vi "9217_Config to Channels.vi"(8 "error in (no error)":errorcluster, 11 "_9217 Config Data":T2={"Conversion Time"=0, "Degree Range"=[], "RTD_Type"=[1], "RTD_A"=[], "RTD_B"=[], "RTD_C"=[], "RTD_Ro"=[]} {"Conversion Time" items=["200 ms", "2.5 ms"]; "Degree Range" items=["Raw Ohms", "Degrees Kelvin", "Degrees Celsius", "Degrees Fahrenheit", "Degrees Rankine"]; "RTD_Type" items=["TCR3851"=1, "TCR3750"=2, "TCR3916"=3, "TCR3920"=4, "TCR3911"=5, "TCR3928"=6, "Custom"=0]}) -> (0 "error out":errorcluster, 2 "Conversion Time":u16(ring) items=["200 ms", "2.5 ms"], 3 "Channels":T1(array[cluster]))   [LabVIEW 2011, in "Modules.lvlib" / "9217.lvclass"]
uses:
  9217.lvclass
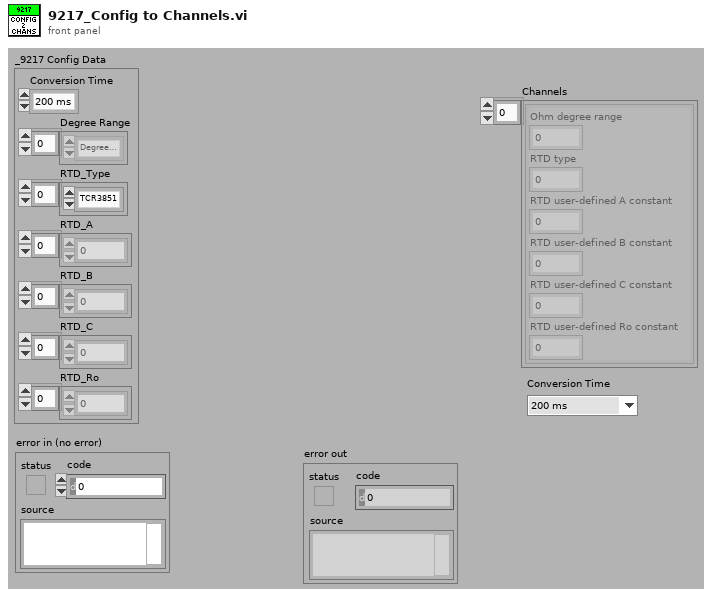
[diagram p1: front panel]
types:
  T1 = cluster{"Ohm degree range":u32, "RTD type":u32, "RTD user-defined A constant":dbl, "RTD user-defined B constant":dbl, "RTD user-defined C constant":dbl, "RTD user-defined Ro constant":dbl}[]
  T2 = cluster{"Conversion Time":u16, "Degree Range":u8[], "RTD_Type":u8[], "RTD_A":dbl[], "RTD_B":dbl[], "RTD_C":dbl[], "RTD_Ro":dbl[]}
  T3 = cluster{"Ohm degree range":u32, "RTD type":u32, "RTD user-defined A constant":dbl, "RTD user-defined B constant":dbl, "RTD user-defined C constant":dbl, "RTD user-defined Ro constant":dbl}
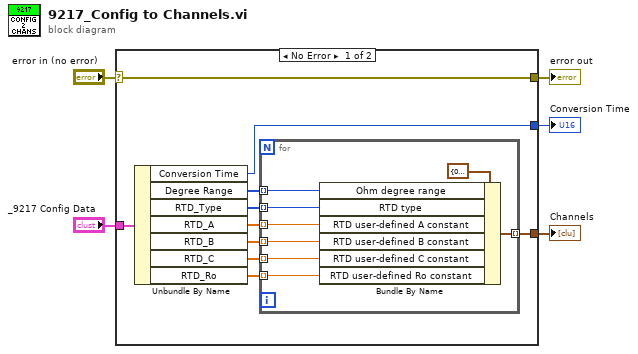
[diagram p0: block diagram]
diagram:
  n1 = case shown="No Error" "error in (no error)" {
    selector: "error in (no error)" -> [w15 w24]
    tunnel: [w15 w24] -> w4
    tunnel: "_9217 Config Data" -> [w14 _]
    tunnel: [w12 _] -> w2
    tunnel: [w6 _] -> w1
    frame No Error {
      n2 = Unbundle By Name(w14) -> ("Conversion Time"=w12:u16, "Degree Range"=w13:u8[], "RTD_Type"=w11:u8[], "RTD_A"=w10:dbl[], "RTD_B"=w9:dbl[], "RTD_C"=w8:dbl[], "RTD_Ro"=w7:dbl[])
      n3 = for {
        tunnel: w13 -> [w22] mode=indexing
        tunnel: w11 -> [w21] mode=indexing
        tunnel: w10 -> [w20] mode=indexing
        tunnel: w9 -> [w19] mode=indexing
        tunnel: w8 -> [w18] mode=indexing
        tunnel: w7 -> [w17] mode=indexing
        tunnel: [w16] -> w6 mode=indexing
        n4 = Bundle By Name(cluster=T3 {"Ohm degree range"=0, "RTD type"=0, "RTD user-defined A constant"=0.0, "RTD user-defined B constant"=0.0, "RTD user-defined C constant"=0.0, "RTD user-defined Ro constant"=0.0} ("Channel"), "Ohm degree range"=w22, "RTD type"=w21, "RTD user-defined A constant"=w20, "RTD user-defined B constant"=w19, "RTD user-defined C constant"=w18, "RTD user-defined Ro constant"=w17) -> (w16:T3)
      }
    }
    frame Error {
    }
  }
  "Channels" <- w1
  "error out" <- w4
  "Conversion Time" <- w2
